vi "FInal.vi"() -> ()   [LabVIEW 2022 SP3]
uses:
  <vilib>/DAQmx/write.llb/DAQmx Write (Digital Bool 1Line 1Point).vi
  <vilib>/DAQmx/create/channels.llb/DAQmx Create Channel (DO-Digital Output).vi
  <vilib>/DAQmx/create/channels.llb/DAQmx Create Channel (AI-Voltage-Basic).vi
  <vilib>/DAQmx/miscellaneous.llb/DAQmx Fill In Error Info.vi
  <vilib>/DAQmx/read.llb/DAQmx Read (Analog 1D DBL NChan 1Samp).vi
panel:
  out "Intensity Waveform":dbl(graph)
  out "Temperature Waveform":dbl(graph)
  in  "stop 2":bool
  in  "VISA Refnum in 3":refnum<visa-resource-name>
  in  "VISA Refnum in 2":refnum<visa-resource-name>
  in  "VISA Refnum in":refnum<visa-resource-name>
  out "Bulb":bool
  out "Fan":bool
  out "Intensity measurement":dbl
  out "Window Open":bool
  out "Motion detection":bool
  out "No Rain":bool
  out "Motion":bool
  out "Valid Intensity":bool
  out "Time":dbl
  in  "Bulb":tag
  in  "Window rotate":tag
  in  "Fan":tag
  out "Temperature":dbl
  out "Tempertaure Indicator":dbl(knob) scale=25.0..35.0
  in  "INPUTS":tag
  in  "Shade":tag
  out "Intensity Indicator":dbl(knob) scale=0.0..1000.0
  in  "stop":bool
  # "SMART WINDOW SYSTEM FOR LIBRARY"
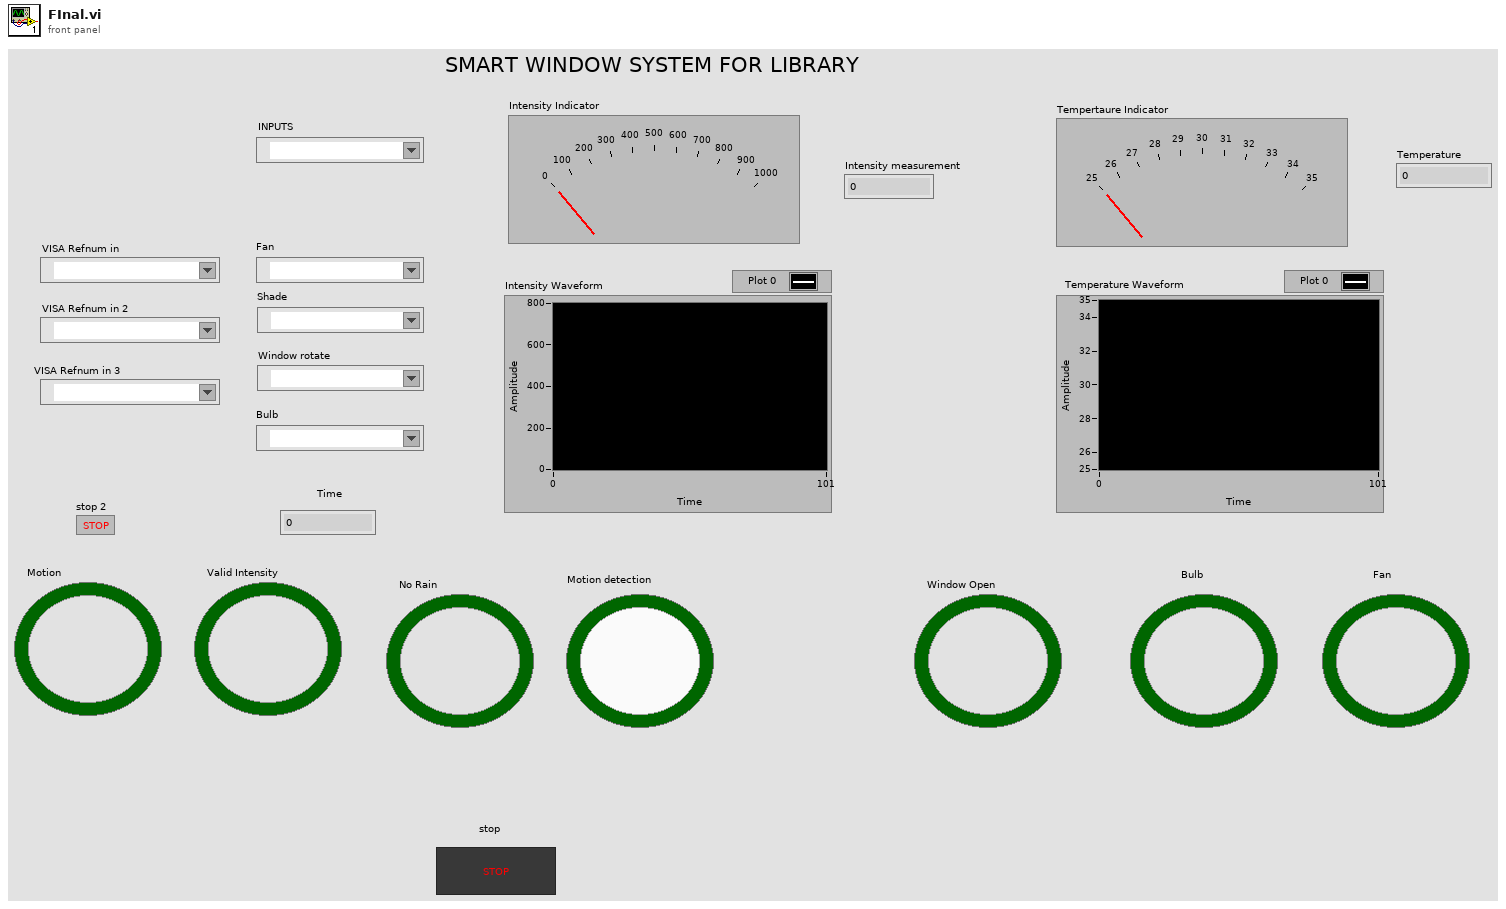
[diagram p1: front panel]
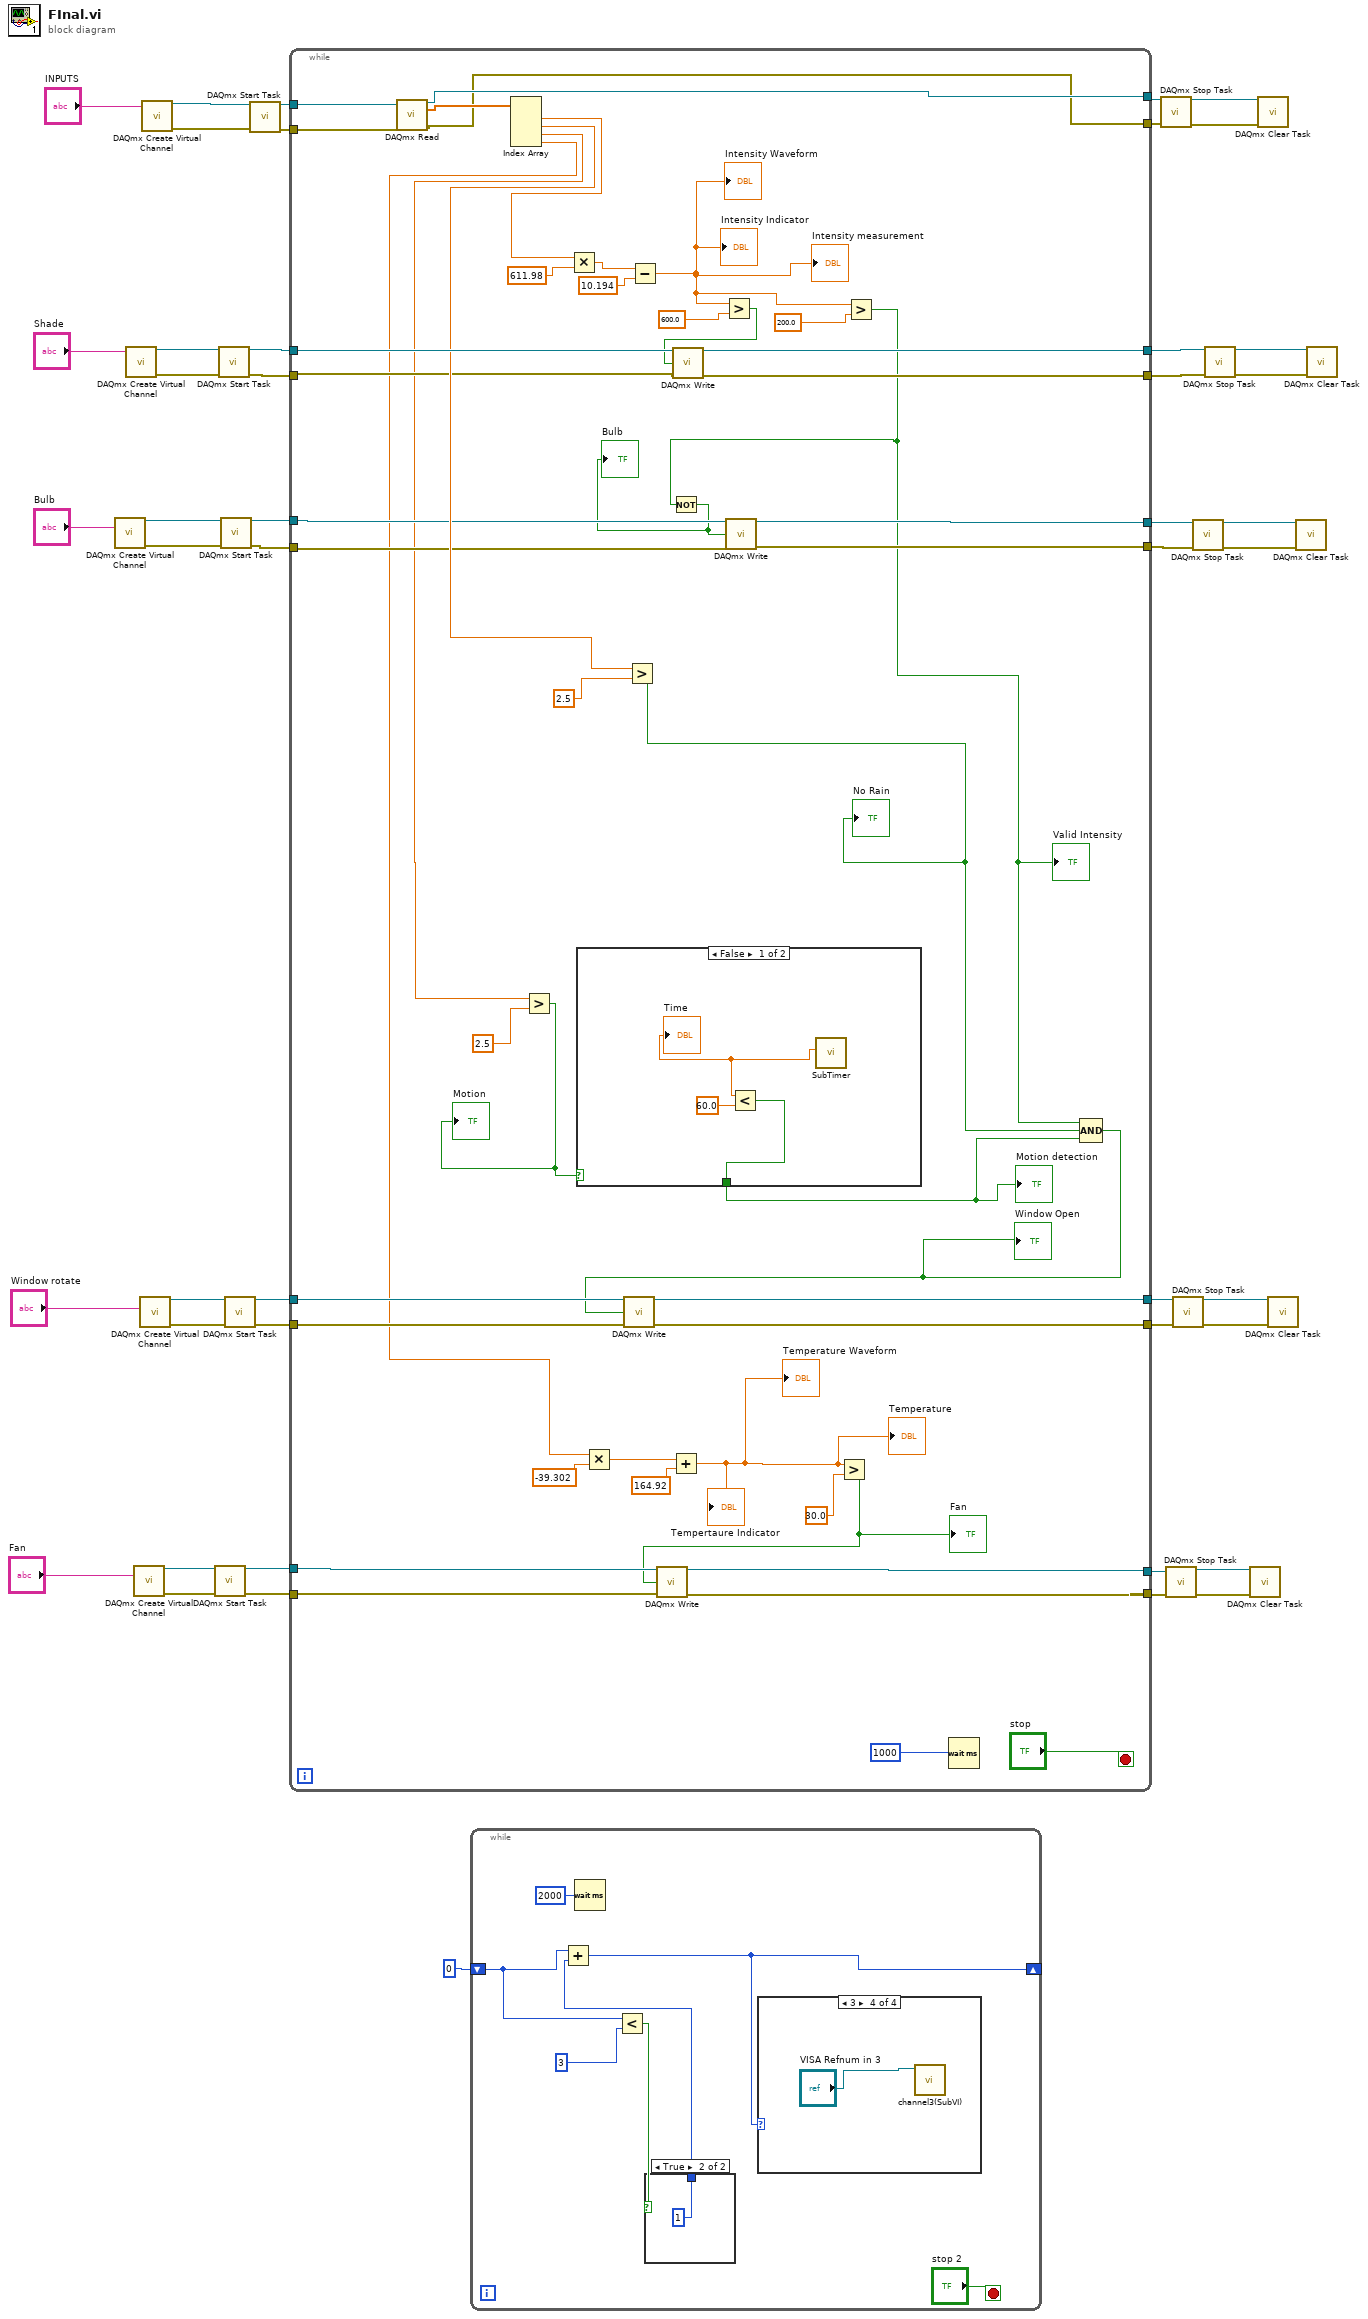
[diagram p0: block diagram]
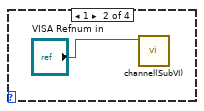
[diagram p3: hidden frame]
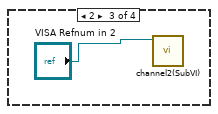
[diagram p4: hidden frame]
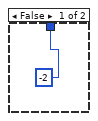
[diagram p5: hidden frame]
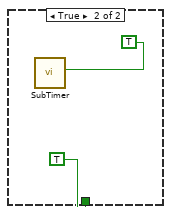
[diagram p6: hidden frame]
diagram:
  n1 = call-poly <vilib>:"DAQmx Create Virtual Channel.vi"("lines"="Bulb") -> ("task out"=w25:refnum<k21>, "error out"=w14:errorcluster)  [unwired: 13 in]
  n2 = call-poly <vilib>:"DAQmx Create Virtual Channel.vi"("lines"="Shade") -> ("task out"=w44:refnum<k21>, "error out"=w17:errorcluster)  [unwired: 13 in]
  n3 = call-poly <vilib>:"DAQmx Create Virtual Channel.vi"("lines"="Fan") -> ("task out"=w36:refnum<k21>, "error out"=w5:errorcluster)  [unwired: 13 in]
  n4 = call-poly <vilib>:"DAQmx Create Virtual Channel.vi"("lines"="Window rotate") -> ("task out"=w31:refnum<k21>, "error out"=w9:errorcluster)  [unwired: 13 in]
  n5 = call-poly <vilib>:"DAQmx Create Virtual Channel.vi"("physical channels"="INPUTS") -> ("task out"=w40:refnum<k21>, "error out"=w21:errorcluster)  [unwired: 13 in]
  n6 = call <vilib>:"DAQmx Start Task.vi"("task/channels in"=w36, "error in"=w5) -> ("task out"=w34:refnum<k21>, "error out"=w4:errorcluster)  [unwired: 12 in]
  n7 = call <vilib>:"DAQmx Start Task.vi"("task/channels in"=w44, "error in"=w17) -> ("task out"=w46:refnum<k21>, "error out"=w16:errorcluster)  [unwired: 12 in]
  n8 = call <vilib>:"DAQmx Start Task.vi"("task/channels in"=w25, "error in"=w14) -> ("task out"=w23:refnum<k21>, "error out"=w13:errorcluster)  [unwired: 12 in]
  n9 = call <vilib>:"DAQmx Start Task.vi"("task/channels in"=w31, "error in"=w9) -> ("task out"=w28:refnum<k21>, "error out"=w8:errorcluster)  [unwired: 12 in]
  n10 = call <vilib>:"DAQmx Start Task.vi"("task/channels in"=w40, "error in"=w21) -> ("task out"=w39:refnum<k21>, "error out"=w20:errorcluster)  [unwired: 12 in]
  n11 = while {
    tunnel: w46 -> [w92]
    tunnel: [w90] -> w42
    tunnel: w39 -> [w86]
    tunnel: w34 -> [w77]
    tunnel: [w76] -> w33
    tunnel: [w74] -> w32
    tunnel: w28 -> [w73]
    tunnel: [w72] -> w27
    tunnel: w23 -> [w60]
    tunnel: [w62] -> w22
    tunnel: w20 -> [w71]
    tunnel: [w70] -> w19
    tunnel: w16 -> [w69]
    tunnel: w13 -> [w67]
    tunnel: [w68] -> w11
    tunnel: [w61] -> w10
    tunnel: w8 -> [w66]
    tunnel: [w65] -> w7
    tunnel: w4 -> [w64]
    tunnel: [w63] -> w3
    stop <- "stop" stop-if-true
    n12 = call-poly <vilib>:"DAQmx Read.vi"("task/channels in"=w86, "error in"=w71) -> ("task out"=w74:refnum<k21>, "data"=w85:dbl[], "error out"=w70:errorcluster)  [unwired: 11 in]
    n13 = Index Array "Index Array"(array=w85) -> (element #1=w83:dbl, element #2=w75:dbl, element #3=w58:dbl, element #4=w50:dbl)  [unwired: 4 in]
    n14 = Greater?(x=w58, y=2.5) -> (0:w56:bool)
    "Motion" <- w56
    n15 = Multiply(x=w83, y=611.98) -> (x*y=w89:dbl)
    n16 = case shown="False" w56 {
      tunnel: [w95 TRUE] -> w54
      frame False {
        n17 = call "SubTimer.vi"() -> ("time"=w97:dbl)  [unwired: 11 in]
        "Time" <- w97
        n18 = Less?(x=w97, y=60.0) -> (x < y?=w95:bool)
      }
      frame True {
        n19 = call "SubTimer.vi"("switch"=TRUE) -> ()  [unwired: 10 in, 1 out]
      }
    }
    "Motion detection" <- w54
    n20 = Multiply(x=w50, y=-39.302) -> (x*y=w80:dbl)
    n21 = Greater?(x=w75, y=2.5) -> (0:w55:bool)
    "No Rain" <- w55
    n22 = Subtract(x=w89, y=10.194) -> (x-y=w47:dbl)
    "Intensity Indicator" <- w47
    "Intensity measurement" <- w47
    "Intensity Waveform" <- w47
    n23 = Add(x=w80, y=164.92) -> (x+y=w49:dbl)
    "Tempertaure Indicator" <- w49
    "Temperature" <- w49
    "Temperature Waveform" <- w49
    n24 = Greater?(x=w47, y=600.0) -> (0:w84:bool)
    n25 = call-poly <vilib>:"DAQmx Write.vi"("task/channels in"=w92, "data"=w84, "error in"=w69) -> ("task out"=w90:refnum<k21>, "error out"=w68:errorcluster)  [unwired: 10 in, 1 out]
    n26 = Greater?(x=w49, y=30.0) -> (0:w51:bool)
    "Fan" <- w51
    n27 = call-poly <vilib>:"DAQmx Write.vi"("task/channels in"=w77, "data"=w51, "error in"=w64) -> ("task out"=w76:refnum<k21>, "error out"=w63:errorcluster)  [unwired: 10 in, 1 out]
    n28 = Greater?(x=w47, y=200.0) -> (0:w57:bool)
    "Valid Intensity" <- w57
    n29 = Not(x=w57) -> (.not. x?=w52:bool)
    "Bulb" <- w52
    n30 = call-poly <vilib>:"DAQmx Write.vi"("task/channels in"=w60, "data"=w52, "error in"=w67) -> ("task out"=w62:refnum<k21>, "error out"=w61:errorcluster)  [unwired: 10 in, 1 out]
    n31 = Wait (ms)(milliseconds to wait=u32 1000 ("millisecond timer value")) -> ()  [unwired: 1 out]
    n32 = Compound Arithmetic op=AND(w57, w55, w54) -> (w53:bool)
    "Window Open" <- w53
    n33 = call-poly <vilib>:"DAQmx Write.vi"("task/channels in"=w73, "data"=w53, "error in"=w66) -> ("task out"=w72:refnum<k21>, "error out"=w65:errorcluster)  [unwired: 10 in, 1 out]
  }
  n34 = while {
    shift-right: [w100] -> _
    shift-left: 0 -> [w105]
    stop <- "stop 2" stop-if-true
    n35 = Wait (ms)(milliseconds to wait=u32 2000) -> ()  [unwired: 1 out]
    n36 = Less?(x=w105, y=3) -> (x < y?=w103:bool)
    n37 = case shown="True" w103 {
      tunnel: [-2 1] -> w102
      frame False {
      }
      frame True {
      }
    }
    n38 = Add(x=w105, y=w102) -> (x+y=w100:i32)
    n39 = case shown="3" w100 {
      frame 0, Default {
      }
      frame 1 {
        n40 = call "channel(SubVI).vi"("VISA Refnum in"="VISA Refnum in") -> ()  [unwired: 11 in]
      }
      frame 2 {
        n41 = call "channel2(SubVI).vi"("VISA Refnum in"="VISA Refnum in 2") -> ()  [unwired: 11 in]
      }
      frame 3 {
        n42 = call "channel3(SubVI).vi"("VISA Refnum in"="VISA Refnum in 3") -> ()  [unwired: 11 in]
      }
    }
  }
  n43 = call <vilib>:"DAQmx Stop Task.vi"("task/channels in"=w32, "error in"=w19) -> ("task out"=w38:refnum<k21>, "error out"=w18:errorcluster)  [unwired: 12 in]
  n44 = call <vilib>:"DAQmx Stop Task.vi"("task/channels in"=w33, "error in"=w3) -> ("task out"=w35:refnum<k21>, "error out"=w2:errorcluster)  [unwired: 12 in]
  n45 = call <vilib>:"DAQmx Stop Task.vi"("task/channels in"=w27, "error in"=w7) -> ("task out"=w29:refnum<k21>, "error out"=w6:errorcluster)  [unwired: 12 in]
  n46 = call <vilib>:"DAQmx Stop Task.vi"("task/channels in"=w22, "error in"=w10) -> ("task out"=w24:refnum<k21>, "error out"=w12:errorcluster)  [unwired: 12 in]
  n47 = call <vilib>:"DAQmx Stop Task.vi"("task/channels in"=w42, "error in"=w11) -> ("task out"=w45:refnum<k21>, "error out"=w15:errorcluster)  [unwired: 12 in]
  n48 = call <vilib>:"DAQmx Clear Task.vi"("task in"=w35, "error in"=w2) -> ()  [unwired: 13 in, 1 out]
  n49 = call <vilib>:"DAQmx Clear Task.vi"("task in"=w38, "error in"=w18) -> ()  [unwired: 13 in, 1 out]
  n50 = call <vilib>:"DAQmx Clear Task.vi"("task in"=w29, "error in"=w6) -> ()  [unwired: 13 in, 1 out]
  n51 = call <vilib>:"DAQmx Clear Task.vi"("task in"=w24, "error in"=w12) -> ()  [unwired: 13 in, 1 out]
  n52 = call <vilib>:"DAQmx Clear Task.vi"("task in"=w45, "error in"=w15) -> ()  [unwired: 13 in, 1 out]
